vi "Calculate High Cost Sector.vi"(9 "Forbidden Bearing (degrees)":dbl, 10 "Compass Bearing (degrees)":dbl) -> (1 "Forbidden Sector (Sectors)":i16)   [LabVIEW 2009]
panel:
  out "Target behind robot?":bool
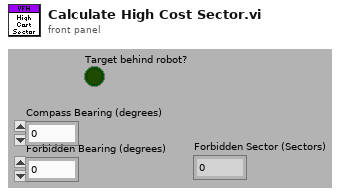
[diagram p1: front panel]
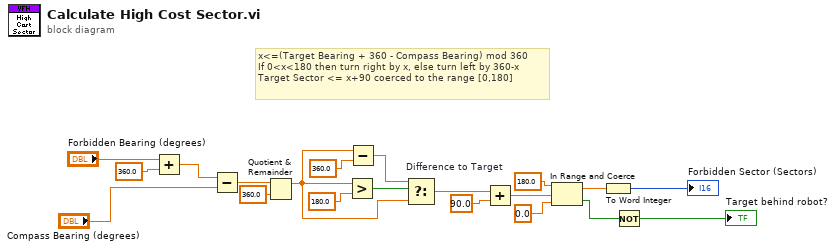
[diagram p0: block diagram]
diagram:
  # "x<=(Target Bearing + 360 - Compass Bearing) mod 360\nIf 0<x<180 then turn right by x, else turn left by 360-x\nTarget Sector <= x+90 coerced to the range [0,180]"
  n1 = Add(x="Forbidden Bearing (degrees)", y=360.0) -> (x+y=w19:dbl)
  n2 = Subtract(x=w19, y="Compass Bearing (degrees)") -> (x-y=w16:dbl)
  n3 = Quotient & Remainder(x=w16, y=360.0) -> (x-y*floor(x/y)=w12:dbl)  [unwired: 1 out]
  n4 = Greater?(x=w12, y=180.0) -> (0:w13:bool)
  n5 = Subtract(x=w12, y=360.0) -> (x-y=w10:dbl)
  n6 = Select "Difference to Target"(t=w10, s=w13, f=w12) -> (s? t:f=w1:dbl)
  n7 = Add(x=w1, y=90.0) -> (x+y=w7:dbl)
  n8 = In Range and Coerce(upper limit=180.0, x=w7, lower limit=0.0) -> (coerced(x)=w4:dbl, In Range?=w3:bool)
  n9 = To Word Integer(number=w4) -> (16bit integer=→"Forbidden Sector (Sectors)":i16)
  n10 = Not(x=w3) -> (.not. x?=→"Target behind robot?":bool)
